vi "convertForFPGA.vi"(8 "error in (no error)":errorcluster, 11 "Modbus in":refnum<class "Modbus.lvclass">) -> (0 "error out":errorcluster, 2 "Data":u16[](array[numeric]), 3 "Modbus out":refnum<class "Modbus.lvclass">)   [LabVIEW 2016, in "RTModbusFPGA.lvlib" / "Modbus.lvclass"]
uses:
  Modbus.lvclass
  Modbus.lvclass/Modbus.ctl
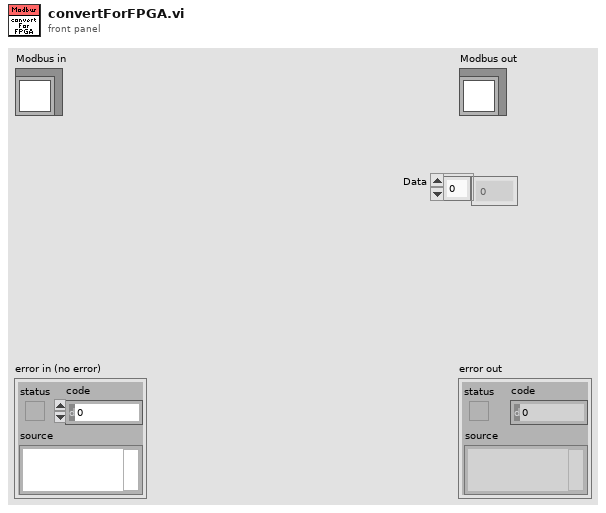
[diagram p1: front panel]
types:
  T1 = typedef "RTModbus.lvlib/TxFrame.ctl" = cluster{"Data":u8[], "WaitForTrigger":bool, "WaitForRx":u32, "TriggerIRQ":bool, "DelayMicroseconds":u16, "DelayMilliseconds":u16, "Timestamp":bool}
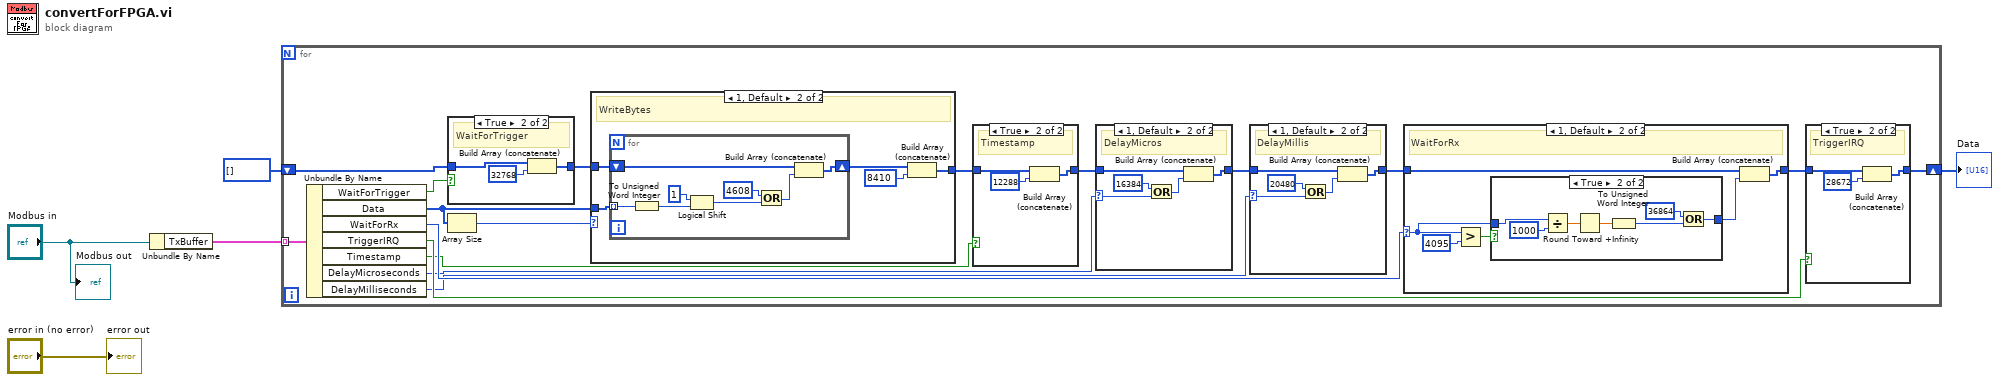
[diagram p0: block diagram]
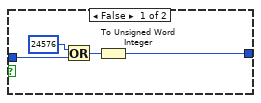
[diagram p8: hidden frame]
diagram:
  n1 = Unbundle By Name("Modbus in") -> ("TxBuffer"=w5:T1[])
  n2 = for {
    tunnel: w5 -> [w22] mode=indexing
    shift-right: [w10] -> w2
    shift-left: u16[] [] -> [w14]
    n3 = Unbundle By Name(w22) -> ("WaitForTrigger"=w11:bool, "Data"=w12:u8[], "WaitForRx"=w21:u32, "TriggerIRQ"=w20:bool, "Timestamp"=w8:bool, "DelayMicroseconds"=w18:u16, "DelayMilliseconds"=w16:u16)
    n4 = case shown="True" w11 {
      tunnel: w14 -> [w75 w76]
      tunnel: [w75 w78] -> w13
      frame False {
      }
      frame True {
        # "WaitForTrigger"
        n5 = Build Array (concatenate)(w76, u16 32768 ("x")) -> (w78:u16[])
      }
    }
    n6 = Array Size(array=w12) -> (size(s)=w15:i32)
    n7 = case shown="1, Default" w15 {
      tunnel: w13 -> [w27 w32]
      tunnel: [w27 w29] -> w7
      tunnel: w12 -> [_ w28]
      frame 0 {
      }
      frame 1, Default {
        # "WriteBytes"
        n8 = for {
          shift-right: [w39] -> w31
          shift-left: w32 -> [w40]
          tunnel: w28 -> [w33] mode=indexing
          n9 = To Unsigned Word Integer(number=w33) -> (unsigned 16bit integer=w38:u16)
          n10 = Logical Shift(y=i16 1, x=w38) -> (x << y=w36:u16)
          n11 = Or(x=u16 4608, y=w36) -> (x .or. y?=w34:u16)
          n12 = Build Array (concatenate)(w40, w34) -> (w39:u16[])
        }
        n13 = Build Array (concatenate)(w31, u16 8410 ("x")) -> (w29:u16[])
      }
    }
    n14 = case shown="True" w8 {
      tunnel: w7 -> [w23 w25]
      tunnel: [w23 w26] -> w6
      frame False {
      }
      frame True {
        # "Timestamp"
        n15 = Build Array (concatenate)(w25, u16 12288 ("x")) -> (w26:u16[])
      }
    }
    n16 = case shown="1, Default" w18 {
      selector: w18 -> [_ w49]
      tunnel: w6 -> [w47 w50]
      tunnel: [w47 w52] -> w17
      frame 0 {
      }
      frame 1, Default {
        # "DelayMicros"
        n17 = Or(x=u16 16384, y=w49) -> (x .or. y?=w51:u16)
        n18 = Build Array (concatenate)(w50, w51) -> (w52:u16[])
      }
    }
    n19 = case shown="1, Default" w16 {
      selector: w16 -> [_ w44]
      tunnel: w17 -> [w41 w45]
      tunnel: [w41 w42] -> w9
      frame 0 {
      }
      frame 1, Default {
        # "DelayMillis"
        n20 = Or(x=u16 20480, y=w44) -> (x .or. y?=w46:u16)
        n21 = Build Array (concatenate)(w45, w46) -> (w42:u16[])
      }
    }
    n22 = case shown="1, Default" w21 {
      selector: w21 -> [_ w59]
      tunnel: w9 -> [w57 w62]
      tunnel: [w57 w63] -> w19
      frame 0 {
      }
      frame 1, Default {
        # "WaitForRx"
        n23 = Greater?(x=w59, y=u32 4095) -> (0:w60:bool)
        n24 = case shown="True" w60 {
          tunnel: w59 -> [w66 w72]
          tunnel: [w64 w73] -> w58
          frame False {
            n25 = Or(x=u16 24576, y=w66) -> (x .or. y?=w65:u32)
            n26 = To Unsigned Word Integer(number=w65) -> (unsigned 16bit integer=w64:u16)
          }
          frame True {
            n27 = Divide(x=w72, y=u32 1000) -> (x/y=w70:dbl)
            n28 = Round Toward +Infinity(x=w70) -> (ceil(x): smallest int >= x=w69:dbl)
            n29 = To Unsigned Word Integer(number=w69) -> (unsigned 16bit integer=w68:u16)
            n30 = Or(x=u16 36864, y=w68) -> (x .or. y?=w73:u16)
          }
        }
        n31 = Build Array (concatenate)(w62, w58) -> (w63:u16[])
      }
    }
    n32 = case shown="True" w20 {
      tunnel: w19 -> [w53 w55]
      tunnel: [w53 w56] -> w10
      frame False {
      }
      frame True {
        # "TriggerIRQ"
        n33 = Build Array (concatenate)(w55, u16 28672 ("x")) -> (w56:u16[])
      }
    }
  }
  "Data" <- w2
  "error out" <- "error in (no error)"
  "Modbus out" <- "Modbus in"
